vi "Radau5_Save Old Value.vi"(10 "Timestep index":i32, 11 "Implicit RK Data In":T1) -> (3 "Implicit RK Data Out":T1)   [LabVIEW 2017, in "NI_DAE.lvlib"]
uses:
  <vilib>/gmath/NI_DAE.lvlib
  <vilib>/gmath/dae.llb/Radau5_Implicit RK Data.ctl
  <vilib>/gmath/dae.llb/Radau5_RK Status.ctl
  <vilib>/Analysis/Matrix/Datatypes/RealMatrix.ctl
  <vilib>/Analysis/Matrix/Datatypes/ComplexMatrix.ctl
  <vilib>/Analysis/Matrix/NI_Matrix.lvlib
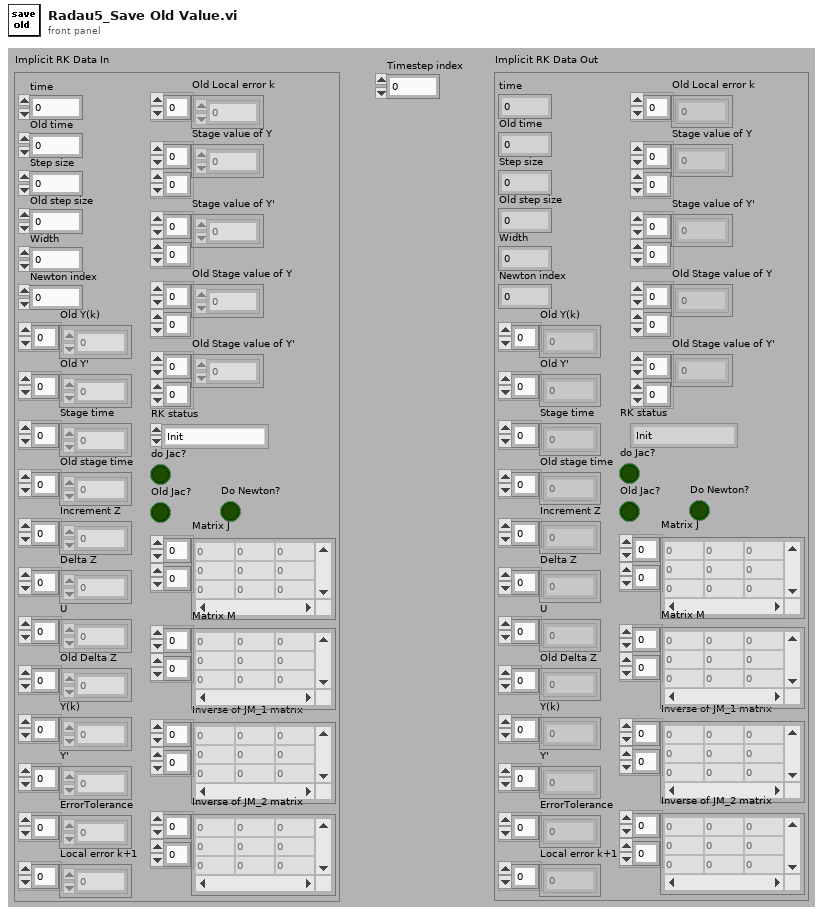
[diagram p1: front panel]
types:
  T1 = typedef "NI_DAE.lvlib/Radau5_Implicit RK Data.ctl" = cluster{"time":dbl, "Old time":dbl, "Step size":dbl, "Old step size":dbl, "Width":i32, "Newton index":i32, "Old Y(k)":dbl[], "Old Y'":dbl[], "Stage time":dbl[], "Old stage time":dbl[], "Increment Z":dbl[], "Delta Z":dbl[], "U":dbl[], "Old Delta Z":dbl[], "Y(k)":dbl[], "Y'":dbl[], "ErrorTolerance":dbl[], "Local error k+1":dbl[], "Old Local error k":dbl[], "Stage value of Y":dbl[][], "Stage value of Y'":dbl[][], "Old Stage value of Y":dbl[][], "Old Stage value of Y'":dbl[][], "RK status":T2, "do Jac?":bool, "Old Jac?":bool, "Do Newton?":bool, "Matrix J":T3, "Matrix M":T3, "Inverse of JM_1 matrix ":T3, "Inverse of JM_2 matrix":T4}
  T2 = typedef "NI_DAE.lvlib/Radau5_RK Status.ctl" = enum16{"Init", "Predict", "Jacobian", "Newton", "error eval y y'", "error eval calc", "next step updata", "reset RK"}
  T3 = typedef "NI_Matrix.lvlib/RealMatrix.ctl" = dbl[][]
  T4 = typedef "NI_Matrix.lvlib/ComplexMatrix.ctl" = cdb[][]
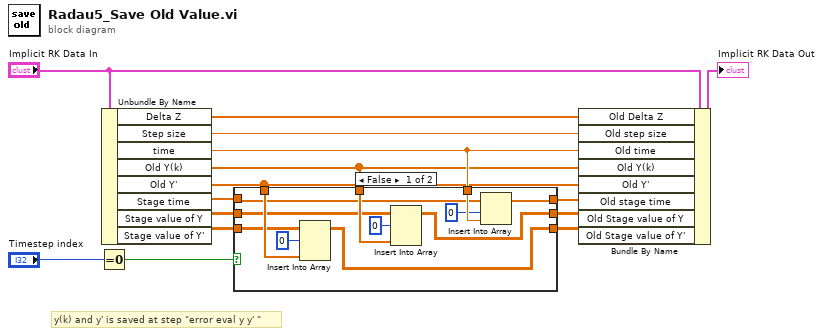
[diagram p0: block diagram]
diagram:
  # "y(k) and y' is saved at step \"error eval y y' \""
  n1 = Equal To 0?(x="Timestep index") -> (x = 0?=w4:bool)
  n2 = Unbundle By Name("Implicit RK Data In") -> ("Delta Z"=w15:dbl[], "Step size"=w12:dbl, "time"=w11:dbl, "Old Y(k)"=w10:dbl[], "Old Y'"=w9:dbl[], "Stage time"=w6:dbl[], "Stage value of Y"=w7:dbl[][], "Stage value of Y'"=w8:dbl[][])
  n3 = case shown="False" w4 {
    tunnel: w11 -> [w27 _]
    tunnel: w10 -> [w24 _]
    tunnel: w9 -> [w22 _]
    tunnel: w8 -> [w21 w28]
    tunnel: w7 -> [w20 w29]
    tunnel: w6 -> [w19 w30]
    tunnel: [w16 w30] -> w3
    tunnel: [w17 w29] -> w2
    tunnel: [w18 w28] -> w1
    frame False {
      n4 = Insert Into Array(array=w21, index (row)=0, new element=w22) -> (w18:dbl[][])  [unwired: 1 in]
      n5 = Insert Into Array(array=w20, index (row)=0, new element=w24) -> (w17:dbl[][])  [unwired: 1 in]
      n6 = Insert Into Array(array=w19, index=0, new element=w27) -> (w16:dbl[])
    }
    frame True {
    }
  }
  n7 = Bundle By Name(cluster="Implicit RK Data In", "Old Delta Z"=w15, "Old step size"=w12, "Old time"=w11, "Old Y(k)"=w10, "Old Y'"=w9, "Old stage time"=w3, "Old Stage value of Y"=w2, "Old Stage value of Y'"=w1) -> (→"Implicit RK Data Out":T1)
